vi "Get Node Info.vi"(8 "error in (no error)":errorcluster, 11 "Node Config in":refnum<class "Node Config.lvclass">) -> (0 "error out":errorcluster, 2 "Info":T1, 3 "Node Config out":refnum<class "Node Config.lvclass">)   [LabVIEW 2020, in "Vecto.lvlib" / "Node Config.lvclass"]
uses:
  Node Config.lvclass
  Node Info.ctl
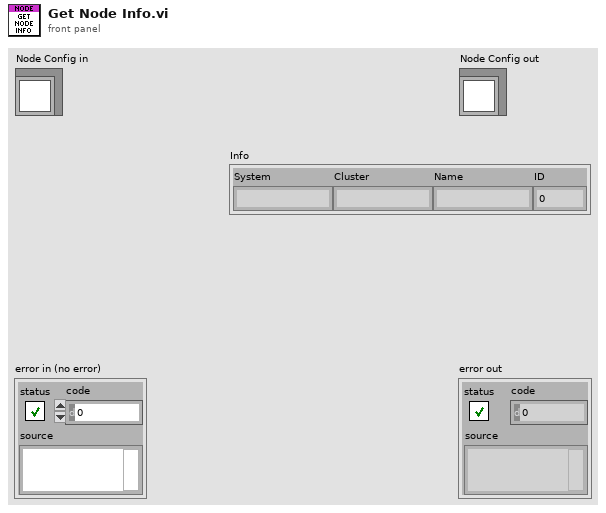
[diagram p1: front panel]
types:
  T1 = typedef "Vecto.lvlib/Node Config.lvclass/Node Info.ctl" = cluster{"System":string, "Cluster":string, "Name":string, "ID":u32}
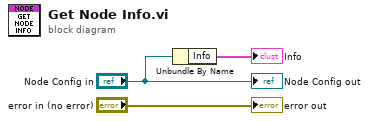
[diagram p0: block diagram]
diagram:
  n1 = Unbundle By Name("Node Config in") -> ("Info"=→"Info":T1)
  "error out" <- "error in (no error)"
  "Node Config out" <- "Node Config in"
